vi "user interface.vi"() -> ()   [LabVIEW 2014]
uses:
  control/FGV User variables.ctl
  control/FGV User states.ctl
  control/FGV Menu buttons user.ctl
  control/FGV Serial Tasks.ctl
panel:
  out "Terminal de linea\n\"QP\"/contacto 2":u32(colorbox)
  out "Brazo - trenza 3":u32(colorbox)
  out "Brazo - contacto 3":u32(colorbox)
  out "Brazo - contacto/Trenza 2":u32(colorbox)
  out "Bimetal - Magneto 2":u32(colorbox)
  out "Terminal - Bimetal 2":u32(colorbox)
  out "Terminal de linea\n\"QP\"/contacto":u32(colorbox)
  out "Brazo - trenza 2":u32(colorbox)
  out "Brazo - contacto 2":u32(colorbox)
  out "Brazo - contacto/Trenza":u32(colorbox)
  out "Bimetal - Magneto":u32(colorbox)
  out "Terminal - Bimetal":u32(colorbox)
  out "Mecanismo":u32(colorbox)
  out "Brazo - trenza":u32(colorbox)
  out "Brazo - contacto":u32(colorbox)
  in  "Linea":u16(ring)=1 items=["Linea 1"=1, "Linea 2"=2, "Linea 3"=3, "Linea 4"=4, "Linea 5"=5]
  in  "Menu":T1
  in  "Soldadora":u16(ring)=1 items=["Brazo - contacto"=1, "Brazo - trenza"=2, "Mecanismo"=3]
  in  "stop":bool
  out "error out":errorcluster
  in  "error in (no error)":errorcluster
  in  "Variables":T2
  # "Linea 1"
  # "Linea 2"
  # "Linea 3"
  # "Linea 4"
  # "Linea 5"
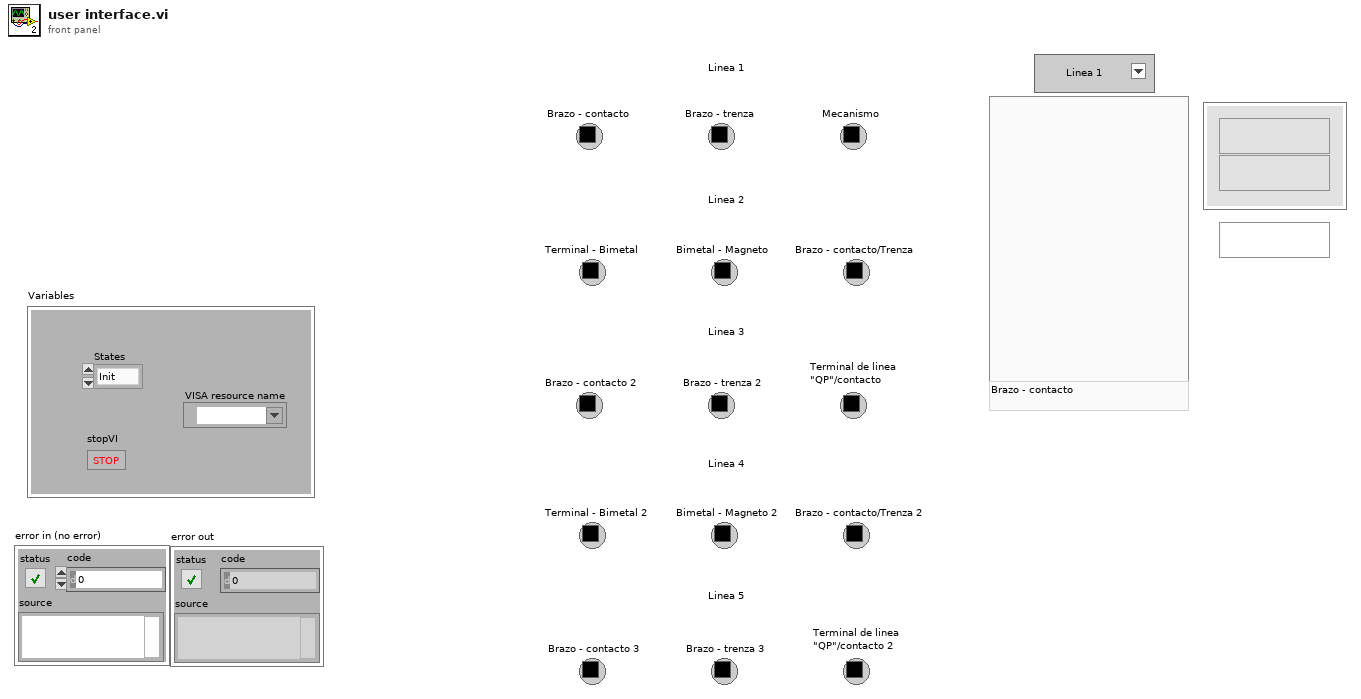
[diagram p1: front panel]
types:
  T1 = typedef "FGV Menu buttons user.ctl" = cluster{"1":bool, "2":bool}
  T2 = typedef "FGV User variables.ctl" = cluster{"States":T3, "stopVI":bool, "VISA resource name":refnum<visa-resource-name>}
  T3 = typedef "FGV User states.ctl" = enum16{"Init", "Idle", "Clean Up", "Exit"}
  T4 = typedef "FGV Serial Tasks.ctl" = enum16{"Open", "Read", "Write", "Close", "Flush"}
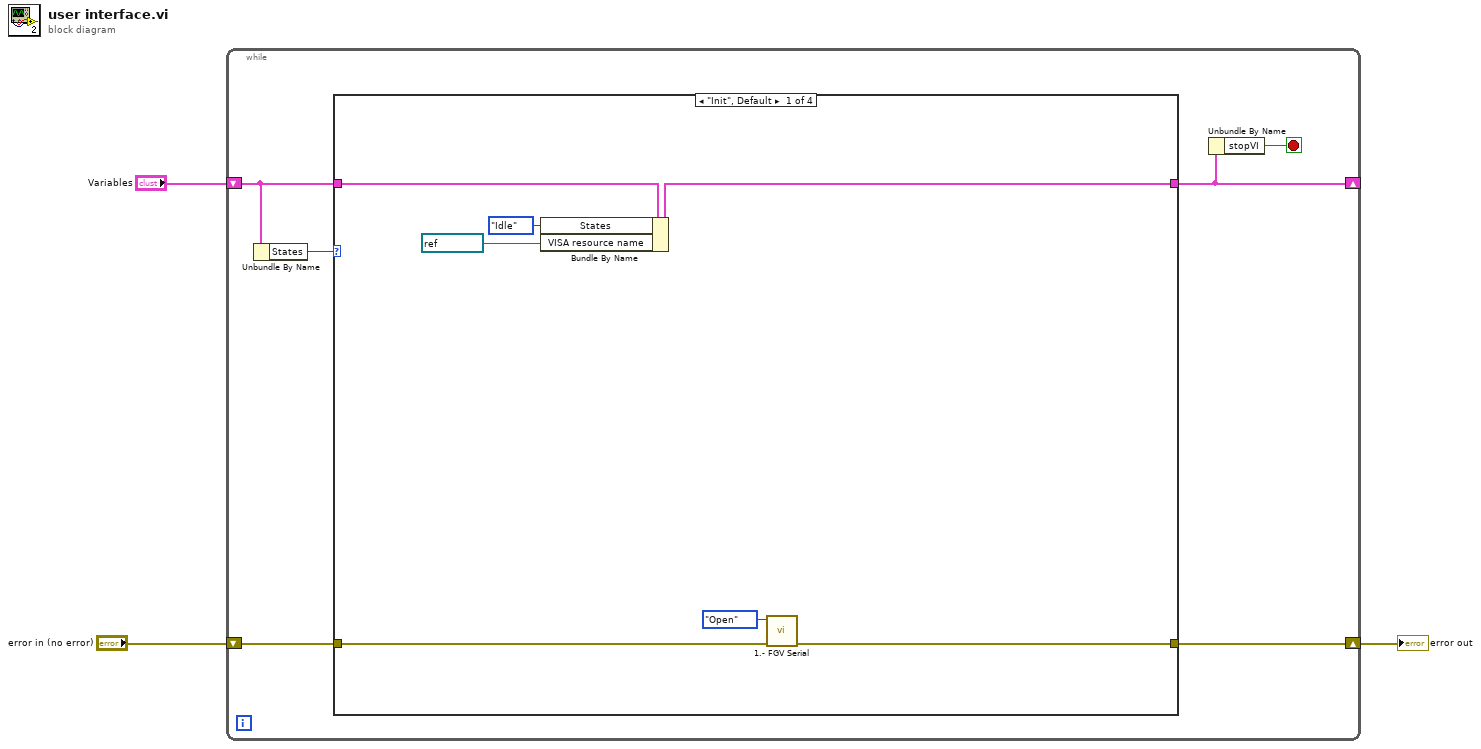
[diagram p0: block diagram]
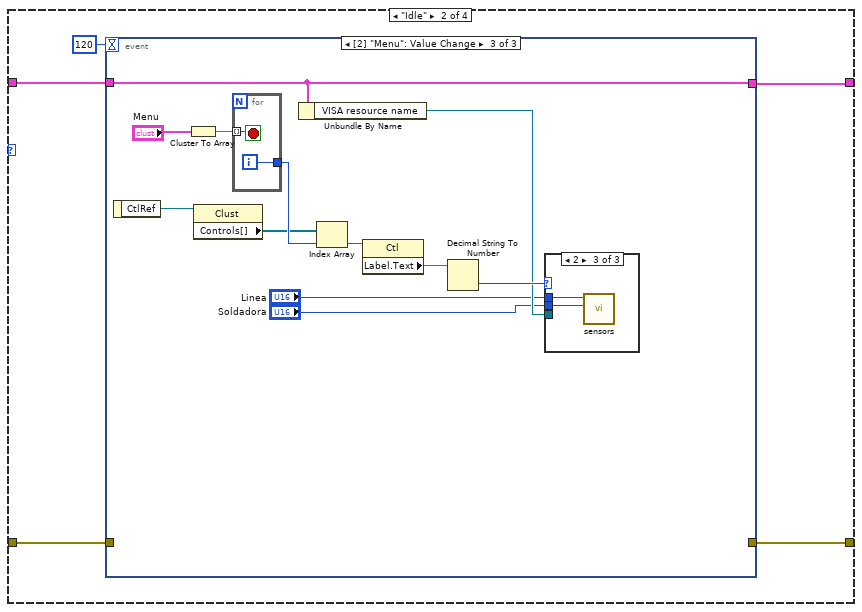
[diagram p2: hidden frame]
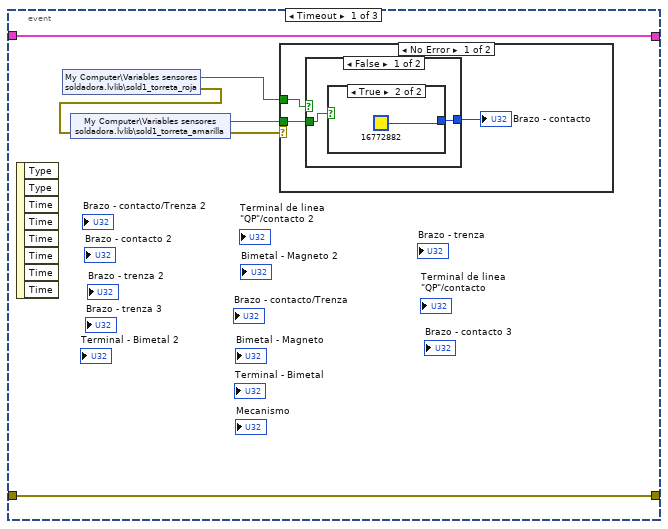
[diagram p3: hidden frame]
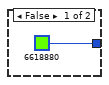
[diagram p4: hidden frame]
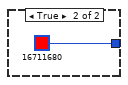
[diagram p5: hidden frame]
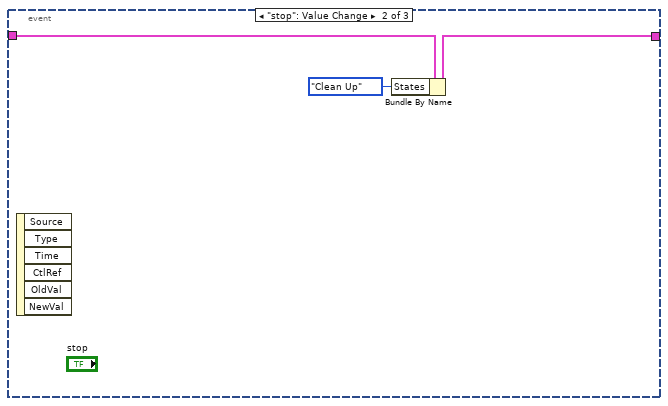
[diagram p7: hidden frame]
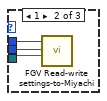
[diagram p9: hidden frame]
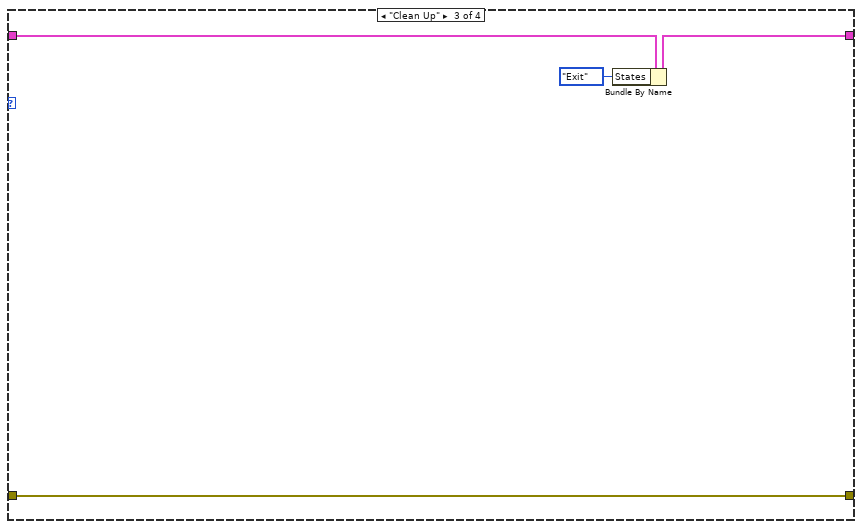
[diagram p10: hidden frame]
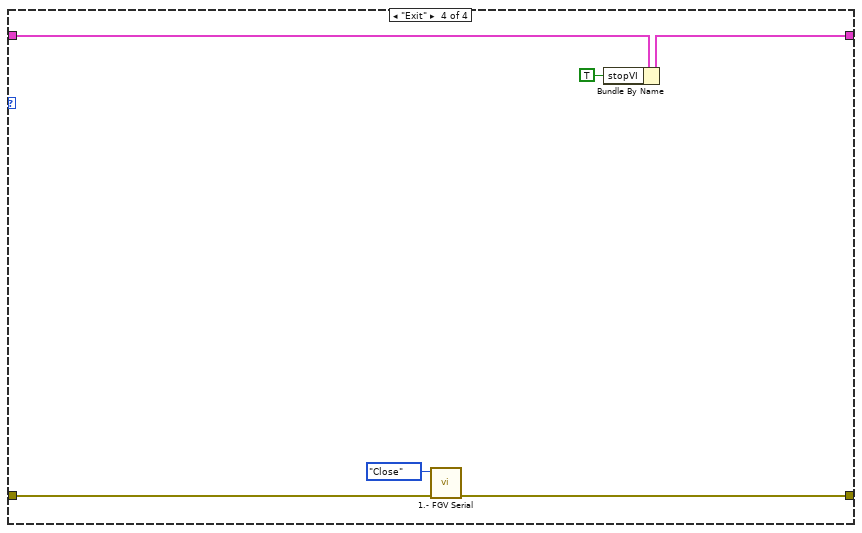
[diagram p11: hidden frame]
diagram:
  n1 = while {
    shift-right: [w5] -> _
    shift-left: "Variables" -> [w9]
    shift-right: [w6] -> w1
    shift-left: "error in (no error)" -> [w7]
    stop <- w4 stop-if-true
    n2 = Unbundle By Name(w9) -> ("States"=w8:T3)
    n3 = case shown="\"Init\", Default" w8 {
      tunnel: w9 -> [w16 w19 w60 w67]
      tunnel: [w15 w18 w59 w66] -> w5
      tunnel: w7 -> [w11 w21 w61 w63]
      tunnel: [w10 w20 w61 w62] -> w6
      frame "Init", Default {
        n4 = Bundle By Name(cluster=w16, "States"=FGV_User_states."Idle", "VISA resource name"=refnum<visa-resource-name> "COM1") -> (w15:T2)
        n5 = call "1.- FGV Serial.vi"("error in (no error)"=w11, "Task"=FGV_Serial_Tasks."Open") -> ("error out"=w10:errorcluster)  [unwired: 7 in, 2 out]
      }
      frame "Idle" {
        n6 = event shown="[2] \"Menu\": Value Change" {
          selector: _ -> [_ _ _]
          dyn-events: _ -> [_ _ _]
          timeout: 120 -> [_ _ _]
          tunnel: [w27 _ _] -> w20
          tunnel: w21 -> [w27 _ _]
          tunnel: w19 -> [w26 w38 w42]
          tunnel: [w26 w37 w42] -> w18
          event Timeout {
            n7 = event-data() -> ()  [unwired: 1 in, 8 out]
            n8 = shared-variable "My Computer\\Variables sensores soldadora.lvlib\\sold1_torreta_roja"() -> (w25:bool, error out=w22:errorcluster)  [unwired: 1 in]
            n9 = shared-variable "My Computer\\Variables sensores soldadora.lvlib\\sold1_torreta_amarilla"(error in=w22) -> (w24:bool, error out=w23:errorcluster)
            n10 = case shown="No Error" w23 {
              tunnel: w24 -> [w30 _]
              tunnel: w25 -> [w29 _]
              frame No Error {
                n11 = case shown="False" w29 {
                  tunnel: w30 -> [w32 _]
                  tunnel: [w31 u32 16711680] -> w28
                  frame False {
                    n12 = case shown="True" w32 {
                      tunnel: [u32 6618880 u32 16772882] -> w31
                      frame False {
                      }
                      frame True {
                      }
                    }
                  }
                  frame True {
                  }
                }
                "Brazo - contacto" <- w28
              }
              frame Error {
              }
            }
          }
          event "stop": Value Change {
            n13 = event-data() -> ()  [unwired: 1 in, 6 out]
            n14 = Bundle By Name(cluster=w38, "States"=FGV_User_states."Clean Up") -> (w37:T2)
          }
          event Value Change {
            n15 = event-data() -> ("CtlRef"=w48:refnum<vi>)  [unwired: 1 in]
            n16 = Cluster To Array(cluster="Menu") -> (array=w49:bool[])
            n17 = property class="Clust"(reference=w48) -> ("Controls[]"=w46:refnum<vi>[])  [unwired: 1 in, 2 out]
            n18 = for {
              tunnel: w49 -> [w57] mode=indexing
              tunnel: [w56] -> w47
              i -> [w56]
              stop <- w57 stop-if-true
            }
            n19 = Unbundle By Name(w42) -> ("VISA resource name"=w41:refnum<visa-resource-name>)
            n20 = Index Array(array=w46, index=w47) -> (element=w45:refnum<vi>)
            n21 = property class="Ctl"(reference=w45) -> ("Label.Text"=w44:string)  [unwired: 1 in, 2 out]
            n22 = Decimal String To Number(string=w44) -> (number=w43:i32)  [unwired: 2 in, 1 out]
            n23 = case shown="2" w43 {
              tunnel: "Linea" -> [_ w52 w55]
              tunnel: "Soldadora" -> [_ w53 w54]
              tunnel: w41 -> [_ w51 _]
              frame 0, Default {
              }
              frame 1 {
                n24 = call "FGV Read-write settings-to-Miyachi.vi"("VISA resource name"=w51, "Soldadora"=w53, "Linea"=w52) -> ()  [unwired: 8 in, 1 out]
              }
              frame 2 {
                n25 = call "sensors.vi"("Soldadora"=w54, "Linea"=w55) -> ()  [unwired: 10 in]
              }
            }
          }
        }
      }
      frame "Clean Up" {
        n26 = Bundle By Name(cluster=w60, "States"=FGV_User_states."Exit") -> (w59:T2)
      }
      frame "Exit" {
        n27 = call "1.- FGV Serial.vi"("error in (no error)"=w63, "Task"=FGV_Serial_Tasks."Close") -> ("error out"=w62:errorcluster)  [unwired: 7 in, 2 out]
        n28 = Bundle By Name(cluster=w67, "stopVI"=TRUE) -> (w66:T2)
      }
    }
    n29 = Unbundle By Name(w5) -> ("stopVI"=w4:bool)
  }
  "error out" <- w1
